vi "Scalar Field copy.vi"() -> ()   [LabVIEW 2017]
uses:
  <vilib>/Utility/sysdir.llb/System Directory Type.ctl
  <instrlib>/tio-labview/TIO Library/TIO Stream Open.vi
  <instrlib>/tio-labview/TIO Library/TIO RPC Send REQuest.vi
  <instrlib>/tio-labview/TIO Library/TIO RPC Blocking.vi
  <instrlib>/tio-labview/Labview Signal Processing/Log Binning.vi
  <instrlib>/tio-labview/TIO Library/TIO RPC Parse Reply.vi
  <instrlib>/tio-labview/TIO Library/TIO RPC Parse Reply Error.vi
  <instrlib>/tio-labview/TIO Library/TIO Data Stream Parse timebase Info.vi
  <instrlib>/tio-labview/TIO Library/TIO Data Stream Parse pstream Info.vi
  <instrlib>/tio-labview/TIO Library/TIO Data Stream Parse dstream Info.vi
  <instrlib>/tio-labview/TIO Library/TIO Serial Port Name Search.vi
  <instrlib>/tio-labview/TIO Library/TIO Stream Write.vi
  <instrlib>/tio-labview/TIO Library/TIO RPC Form Request.vi
  <instrlib>/tio-labview/TIO Library/TIO Stream Read.vi
  <instrlib>/tio-labview/Labview Signal Processing/Log Range.vi
  <instrlib>/tio-labview/TIO Library/TIO SLIP Serial Write.vi
  <instrlib>/tio-labview/TIO Library/TIO Form Packet.vi
  <instrlib>/tio-labview/TIO Library/TIO Parse Packet.vi
  <instrlib>/tio-labview/TIO Library/TIO SLIP Serial Read.vi
  <instrlib>/tio-labview/TIO Library/TIO SLIP Encode.vi
  <instrlib>/tio-labview/TIO Library/TIO Serial Checksum CRC32.vi
  <vilib>/Utility/tcp.llb/UDP Multicast Open.vi
  <vilib>/Utility/tcp.llb/UDP Multicast Read-Write Open.vi
  <instrlib>/tio-labview/TIO Library/TIO Serial Port Discovery.vi
  <vilib>/Instr/_visa.llb/VISA Configure Serial Port (Instr).vi
  <vilib>/Analysis/6fits.llb/General Polynomial Fit.vi
  <vilib>/measure/maspectr.llb/FFT Power Spectrum and PSD.vi
  <vilib>/measure/maspectr.llb/FFT Power Spectrum and PSD for 1 Chan.vi
  <instrlib>/tio-labview/TIO Library/TIO Stream Read Non-blocking.vi
panel:
  out "Signal":u8(slide) scale=0.0..256.0
  out "Status":T1(ring)
  in  "Reset":bool
  in  "URL":refnum<visa-resource-name>="tcp://localhost"
  in  "Quit":bool
  in  "Duration":dbl[unit]=1000.0
  out "A":T2(graph)
  in  "Log?":bool
  in  "Path":path
  in  "Clear C":bool
  in  "Save C":bool
  in  "Clear B":bool
  in  "Save B":bool
  in  "Clear A":bool
  in  "Save A":bool
  in  "Bin":bool=TRUE
  out "PSD":T3(graph)
  out "ID":string="Twinleaf VM4 R4"
  # "Field"
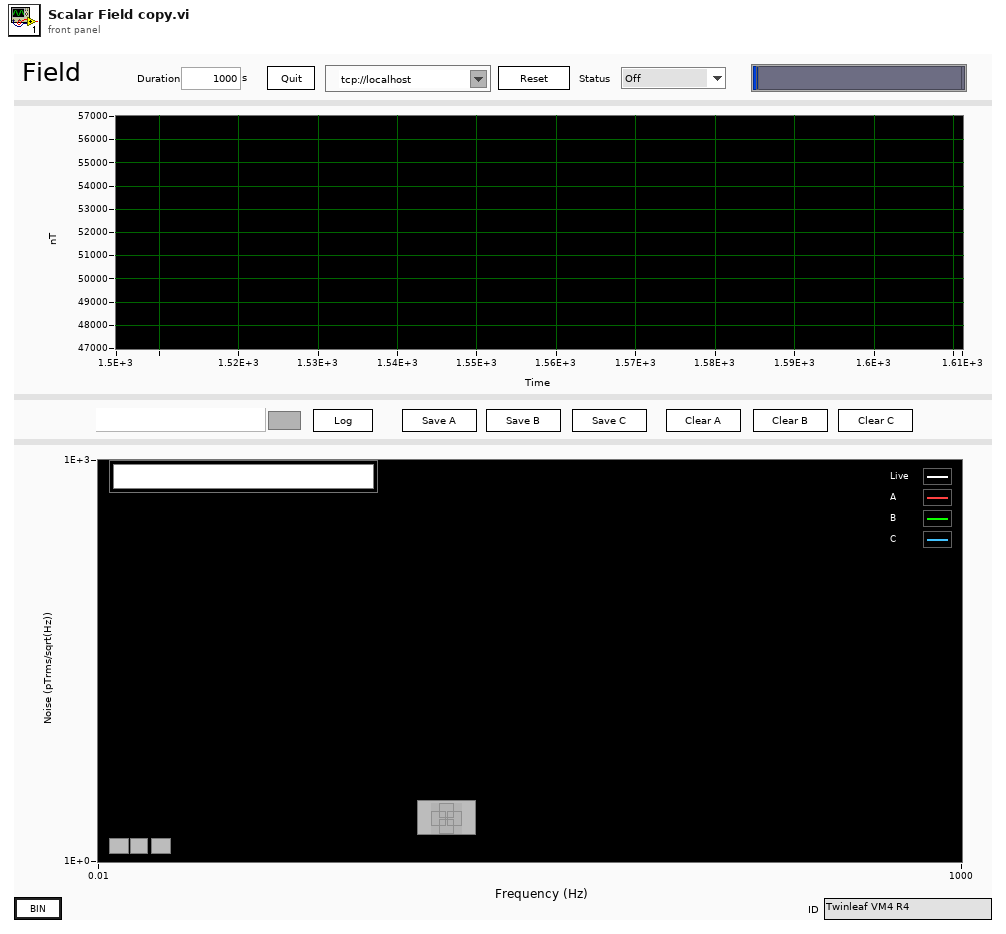
[diagram p1: front panel]
types:
  T1 = enum16{"Off", "Heating", "Laser", "Spin", "Locked"}
  T2 = cluster{"start":dbl, "dt":dbl, "Timeseries":dbl[]}
  T3 = cluster{"Frequencies Binned":dbl[], "Spectrum Binned":dbl[]}[]
  T4 = cluster{"Awaiting REP":bool, "REQ ID":u32, "dstreams in":cluster{"id":u16, "timebase id":u16, "period":u32, "offset":u32, "sample number":u64, "total components":u16, "flags":u16, "components":cluster{"pstream id":u16, "flags":u16, "period":u32, "offset":u32}[]}[], "pstreams":cluster{"id":u16, "timebase_id":u16, "period":u32, "offset":u32, "fmt":i32, "flags":u16, "channels":u16, "type":u8, "name":string, "column names":string[], "title":string, "units":string}[], "timebases":cluster{"id":u16, "source":u16, "epoch":u32, "start time":u32, "period numerator (µs)":i32, "period denominator (µs)":u16, "flags":u16, "stability":u8, "source id":string}[]}
  T5 = typedef "System Directory Type.ctl" = i32
  T6 = cluster{"TS Connection":cluster{"Type":enum16{"Serial", "TCP", "UDP", "mUDP"}, "URL":refnum<visa-resource-name>, "TO":u32, "Addr":u32, "Port":i32, "TCP":refnum<k5>, "UDP":refnum<k16>, "Route":string}, "REQ":refnum<queue>, "REP":refnum<queue>}
  T7 = cluster{"start":dbl, "dt":dbl, "Timeseries":sgl[][]}
  T8 = cluster{"dstream ID":u16, "Sample Number":u32, "Raw Data":string}
  T9 = cluster{"TC Connection":cluster{"Type":enum16{"Serial", "TCP", "UDP", "mUDP"}, "URL":refnum<visa-resource-name>, "TO":u32, "Addr":u32, "Port":i32, "TCP":refnum<k5>, "UDP":refnum<k16>, "Route":string}, "REQ":refnum<queue>, "REP":refnum<queue>}
  T10 = cluster{"start":dbl, "dt":dbl, "Timeseries":dbl[][]}
  T11 = cluster{"Name":string, "Waveform":cluster{"start":dbl, "dt":dbl, "Timeseries":dbl[][]}}[]
  T12 = cluster{"Frequencies Binned":dbl[], "Spectrum Binned":dbl[]}
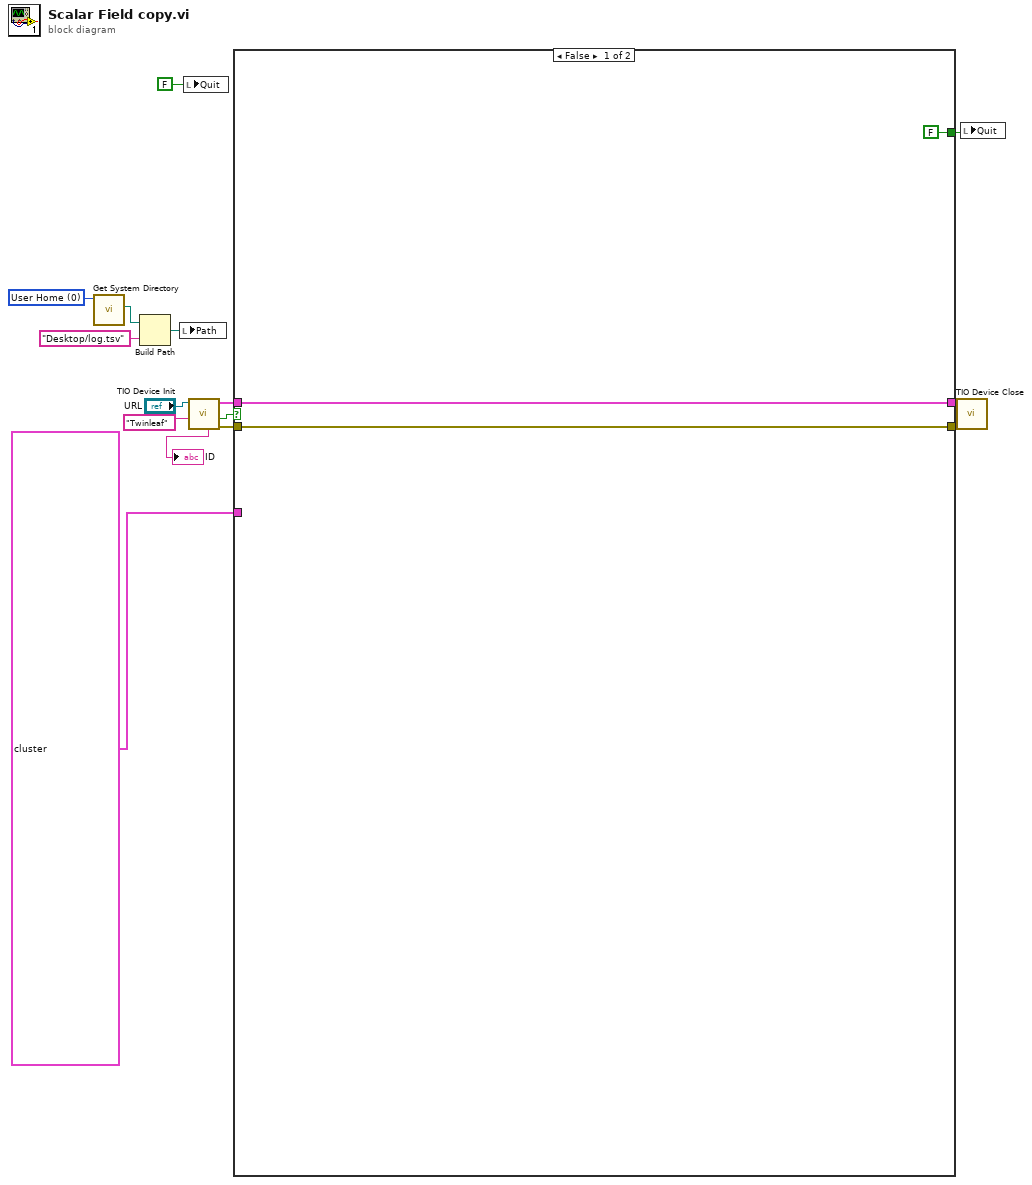
[diagram p0: block diagram]
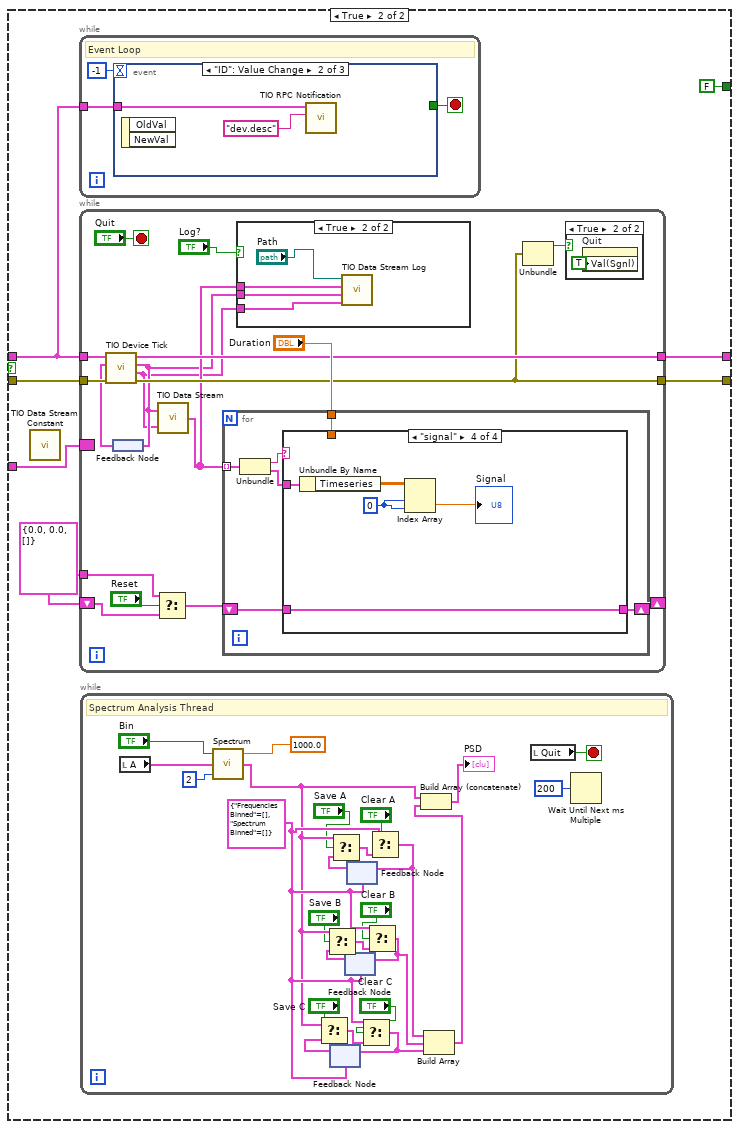
[diagram p2: hidden frame]
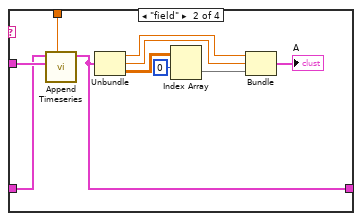
[diagram p6: hidden frame]
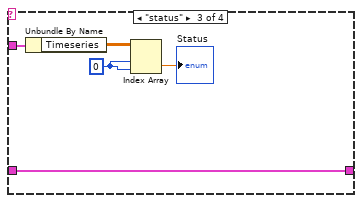
[diagram p7: hidden frame]
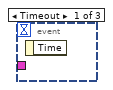
[diagram p8: hidden frame]
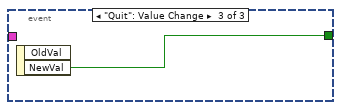
[diagram p9: hidden frame]
diagram:
  w8 = T5 0 items=["User Home"=0, "User Desktop"=1, "User Documents"=2, "User Application Data"=3, "User Preferences"=4, "User Temporary"=5, "Public Documents"=6, "Public Application Data"=7, "Public Preferences"=8, "Public Cache"=13, "System Core Libraries"=9, "System Installed Libraries"=10, "Application Files"=11, "Boot Volume Root"=12] ("system directory type")
  n1 = call <vilib>:"Get System Directory.vi"("system directory type"=w8) -> ("system directory"=w7:path)  [unwired: 10 in]
  n2 = Build Path(base path=w7, name or relative path="Desktop/log.tsv") -> (appended path=w5:path)
  n3 = local write "Path"(w5) -> ()
  n4 = local write "Quit"(FALSE ("Kill")) -> ()
  n5 = call <instrlib>:"TIO Device Init.vi"("ID"="Twinleaf" ("Prefix"), "URL"="URL") -> ("error out"=w14:errorcluster, "Connected"=w3:bool, "TIO"=w15:T6, "ID Verified"=→"ID":string)  [unwired: 5 in, 1 out]
  n6 = case shown="False" w3 {
    tunnel: w15 -> [w18 w24]
    tunnel: w14 -> [w17 w25]
    tunnel: [w17 w22] -> w10
    tunnel: [w18 w21] -> w9
    tunnel: T4 {"Awaiting REP"=FALSE, "REQ ID"=500, "dstreams in"=[{"id"=0, "timebase id"=1, "period"=16, "offset"=0, "sample number"=10656, "total components"=6, "flags"=1, "components"=[{"pstream id"=0, "flags"=0, "period"=1, "offset"=0}, {"pstream id"=1, "flags"=1, "period"=1, "offset"=0}, {"pstream id"=32770, "flags"=0, "period"=8, "offset"=0}, {"pstream id"=32772, "flags"=0, "period"=8, "offset"=0}, {"pstream id"=32774, "flags"=1, "period"=64, "offset"=0}, {"pstream id"=2, "flags"=1, "period"=64, "offset"=0}]}, {"id"=0, "timebase id"=0, "period"=0, "offset"=0, "sample number"=0, "total components"=0, "flags"=0, "components"=[]}, {"id"=0, "timebase id"=0, "period"=0, "offset"=0, "sample number"=0, "total components"=0, "flags"=0, "components"=[]}, {"id"=0, "timebase id"=0, "period"=0, "offset"=0, "sample number"=0, "total components"=0, "flags"=0, "components"=[]}, {"id"=0, "timebase id"=0, "period"=0, "offset"=0, "sample number"=0, "total components"=0, "flags"=0, "components"=[]}, {"id"=0, "timebase id"=0, "period"=0, "offset"=0, "sample number"=0, "total components"=0, "flags"=0, "components"=[]}, {"id"=0, "timebase id"=0, "period"=0, "offset"=0, "sample number"=0, "total components"=0, "flags"=0, "components"=[]}, {"id"=0, "timebase id"=0, "period"=0, "offset"=0, "sample number"=0, "total components"=0, "flags"=0, "components"=[]}, {"id"=0, "timebase id"=0, "period"=0, "offset"=0, "sample number"=0, "total components"=0, "flags"=0, "components"=[]}, {"id"=0, "timebase id"=0, "period"=0, "offset"=0, "sample number"=0, "total components"=0, "flags"=0, "components"=[]}, {"id"=0, "timebase id"=0, "period"=0, "offset"=0, "sample number"=0, "total components"=0, "flags"=0, "components"=[]}, {"id"=0, "timebase id"=0, "period"=0, "offset"=0, "sample number"=0, "total components"=0, "flags"=0, "components"=[]}, {"id"=0, "timebase id"=0, "period"=0, "offset"=0, "sample number"=0, "total components"=0, "flags"=0, "components"=[]}, {"id"=0, "timebase id"=0, "period"=0, "offset"=0, "sample number"=0, "total components"=0, "flags"=0, "components"=[]}, {"id"=0, "timebase id"=0, "period"=0, "offset"=0, "sample number"=0, "total components"=0, "flags"=0, "components"=[]}, {"id"=0, "timebase id"=0, "period"=0, "offset"=0, "sample number"=0, "total components"=0, "flags"=0, "components"=[]}, {"id"=0, "timebase id"=0, "period"=0, "offset"=0, "sample number"=0, "total components"=0, "flags"=0, "components"=[]}, {"id"=0, "timebase id"=0, "period"=0, "offset"=0, "sample number"=0, "total components"=0, "flags"=0, "components"=[]}, {"id"=0, "timebase id"=0, "period"=0, "offset"=0, "sample number"=0, "total components"=0, "flags"=0, "components"=[]}, {"id"=0, "timebase id"=0, "period"=0, "offset"=0, "sample number"=0, "total components"=0, "flags"=0, "components"=[]}, {"id"=0, "timebase id"=0, "period"=0, "offset"=0, "sample number"=0, "total components"=0, "flags"=0, "components"=[]}, {"id"=0, "timebase id"=0, "period"=0, "offset"=0, "sample number"=0, "total components"=0, "flags"=0, "components"=[]}, {"id"=0, "timebase id"=0, "period"=0, "offset"=0, "sample number"=0, "total components"=0, "flags"=0, "components"=[]}, {"id"=0, "timebase id"=0, "period"=0, "offset"=0, "sample number"=0, "total components"=0, "flags"=0, "components"=[]}, {"id"=0, "timebase id"=0, "period"=0, "offset"=0, "sample number"=0, "total components"=0, "flags"=0, "components"=[]}, {"id"=0, "timebase id"=0, "period"=0, "offset"=0, "sample number"=0, "total components"=0, "flags"=0, "components"=[]}, {"id"=0, "timebase id"=0, "period"=0, "offset"=0, "sample number"=0, "total components"=0, "flags"=0, "components"=[]}, {"id"=0, "timebase id"=0, "period"=0, "offset"=0, "sample number"=0, "total components"=0, "flags"=0, "components"=[]}, {"id"=0, "timebase id"=0, "period"=0, "offset"=0, "sample number"=0, "total components"=0, "flags"=0, "components"=[]}, {"id"=0, "timebase id"=0, "period"=0, "offset"=0, "sample number"=0, "total components"=0, "flags"=0, "components"=[]}, {"id"=0, "timebase id"=0, "period"=0, "offset"=0, "sample number"=0, "total components"=0, "flags"=0, "components"=[]}, {"id"=0, "timebase id"=0, "period"=0, "offset"=0, "sample number"=0, "total components"=0, "flags"=0, "components"=[]}], "pstreams"=[{"id"=0, "timebase_id"=1, "period"=8, "offset"=0, "fmt"=-1, "flags"=0, "channels"=1, "type"=66, "name"="field", "column names"=["B"], "title"="Magnetic field", "units"="nT"}, {"id"=1, "timebase_id"=0, "period"=1, "offset"=0, "fmt"=-1, "flags"=0, "channels"=1, "type"=16, "name"="signal", "column names"=[""], "title"="Signal", "units"=""}, {"id"=2, "timebase_id"=0, "period"=1, "offset"=0, "fmt"=-1, "flags"=0, "channels"=1, "type"=16, "name"="status", "column names"=[""], "title"="Status", "units"=""}, {"id"=0, "timebase_id"=0, "period"=0, "offset"=0, "fmt"=0, "flags"=0, "channels"=0, "type"=0, "name"="", "column names"=[], "title"="", "units"=""}, {"id"=0, "timebase_id"=0, "period"=0, "offset"=0, "fmt"=0, "flags"=0, "channels"=0, "type"=0, "name"="", "column names"=[], "title"="", "units"=""}, {"id"=0, "timebase_id"=0, "period"=0, "offset"=0, "fmt"=0, "flags"=0, "channels"=0, "type"=0, "name"="", "column names"=[], "title"="", "units"=""}, {"id"=0, "timebase_id"=0, "period"=0, "offset"=0, "fmt"=0, "flags"=0, "channels"=0, "type"=0, "name"="", "column names"=[], "title"="", "units"=""}, {"id"=0, "timebase_id"=0, "period"=0, "offset"=0, "fmt"=0, "flags"=0, "channels"=0, "type"=0, "name"="", "column names"=[], "title"="", "units"=""}, {"id"=0, "timebase_id"=0, "period"=0, "offset"=0, "fmt"=0, "flags"=0, "channels"=0, "type"=0, "name"="", "column names"=[], "title"="", "units"=""}, {"id"=0, "timebase_id"=0, "period"=0, "offset"=0, "fmt"=0, "flags"=0, "channels"=0, "type"=0, "name"="", "column names"=[], "title"="", "units"=""}, {"id"=0, "timebase_id"=0, "period"=0, "offset"=0, "fmt"=0, "flags"=0, "channels"=0, "type"=0, "name"="", "column names"=[], "title"="", "units"=""}, {"id"=0, "timebase_id"=0, "period"=0, "offset"=0, "fmt"=0, "flags"=0, "channels"=0, "type"=0, "name"="", "column names"=[], "title"="", "units"=""}, {"id"=0, "timebase_id"=0, "period"=0, "offset"=0, "fmt"=0, "flags"=0, "channels"=0, "type"=0, "name"="", "column names"=[], "title"="", "units"=""}, {"id"=0, "timebase_id"=0, "period"=0, "offset"=0, "fmt"=0, "flags"=0, "channels"=0, "type"=0, "name"="", "column names"=[], "title"="", "units"=""}, {"id"=0, "timebase_id"=0, "period"=0, "offset"=0, "fmt"=0, "flags"=0, "channels"=0, "type"=0, "name"="", "column names"=[], "title"="", "units"=""}, {"id"=0, "timebase_id"=0, "period"=0, "offset"=0, "fmt"=0, "flags"=0, "channels"=0, "type"=0, "name"="", "column names"=[], "title"="", "units"=""}, {"id"=32768, "timebase_id"=1, "period"=8, "offset"=0, "fmt"=-1, "flags"=0, "channels"=1, "type"=66, "name"="_field.raw", "column names"=["B"], "title"="Magnetic field", "units"="nT"}, {"id"=32769, "timebase_id"=1, "period"=8, "offset"=0, "fmt"=-1, "flags"=0, "channels"=3, "type"=66, "name"="_spin.raw", "column names"=["measure", "reference", "output"], "title"="Spin lock", "units"=""}, {"id"=32770, "timebase_id"=1, "period"=8, "offset"=0, "fmt"=-1, "flags"=0, "channels"=3, "type"=66, "name"="spin", "column names"=["measure", "reference", "output"], "title"="Spin lock", "units"=""}, {"id"=32771, "timebase_id"=1, "period"=2, "offset"=0, "fmt"=-1, "flags"=0, "channels"=3, "type"=66, "name"="_laser.raw", "column names"=["measure", "reference", "output"], "title"="Laser lock", "units"=""}, {"id"=32772, "timebase_id"=1, "period"=2, "offset"=0, "fmt"=-1, "flags"=0, "channels"=3, "type"=66, "name"="laser", "column names"=["measure", "reference", "output"], "title"="Laser lock", "units"=""}, {"id"=32773, "timebase_id"=2, "period"=1, "offset"=0, "fmt"=-1, "flags"=0, "channels"=3, "type"=66, "name"="_therm.raw", "column names"=["measure", "reference", "output"], "title"="Cell temperature", "units"="°C"}, {"id"=32774, "timebase_id"=2, "period"=1, "offset"=0, "fmt"=-1, "flags"=0, "channels"=3, "type"=66, "name"="therm", "column names"=["measure", "reference", "output"], "title"="Cell temperature", "units"="°C"}, {"id"=32775, "timebase_id"=0, "period"=1, "offset"=0, "fmt"=-1, "flags"=0, "channels"=1, "type"=66, "name"="_cpu.raw", "column names"=[""], "title"="CPU load", "units"="%"}, {"id"=32776, "timebase_id"=0, "period"=1, "offset"=0, "fmt"=-1, "flags"=0, "channels"=1, "type"=66, "name"="cpu", "column names"=[""], "title"="CPU load", "units"="%"}, {"id"=0, "timebase_id"=0, "period"=0, "offset"=0, "fmt"=0, "flags"=0, "channels"=0, "type"=0, "name"="", "column names"=[], "title"="", "units"=""}, {"id"=0, "timebase_id"=0, "period"=0, "offset"=0, "fmt"=0, "flags"=0, "channels"=0, "type"=0, "name"="", "column names"=[], "title"="", "units"=""}, {"id"=0, "timebase_id"=0, "period"=0, "offset"=0, "fmt"=0, "flags"=0, "channels"=0, "type"=0, "name"="", "column names"=[], "title"="", "units"=""}, {"id"=0, "timebase_id"=0, "period"=0, "offset"=0, "fmt"=0, "flags"=0, "channels"=0, "type"=0, "name"="", "column names"=[], "title"="", "units"=""}, {"id"=0, "timebase_id"=0, "period"=0, "offset"=0, "fmt"=0, "flags"=0, "channels"=0, "type"=0, "name"="", "column names"=[], "title"="", "units"=""}, {"id"=0, "timebase_id"=0, "period"=0, "offset"=0, "fmt"=0, "flags"=0, "channels"=0, "type"=0, "name"="", "column names"=[], "title"="", "units"=""}, {"id"=0, "timebase_id"=0, "period"=0, "offset"=0, "fmt"=0, "flags"=0, "channels"=0, "type"=0, "name"="", "column names"=[], "title"="", "units"=""}], "timebases"=[{"id"=0, "source"=513, "epoch"=0, "start time"=0, "period numerator (µs)"=100000000, "period denominator (µs)"=1000, "flags"=0, "stability"=1, "source id"="\u0000\u0000\u0000\u0000\u0000À\u0001\u0000\u0000\u0000@\u0000\u001f\u0000\u0011P6W462 "}, {"id"=1, "source"=513, "epoch"=187833658, "start time"=0, "period numerator (µs)"=312500, "period denominator (µs)"=1000, "flags"=0, "stability"=1, "source id"="\u0000\u0000\u0000¬Å'7\u0001\u0000\u0000\u0000@\u0000\u001f\u0000\u0011P6W462 "}, {"id"=2, "source"=513, "epoch"=62622070, "start time"=0, "period numerator (µs)"=125000000, "period denominator (µs)"=1000, "flags"=0, "stability"=1, "source id"="\u0000\u0000\u0000\nף;\u0001\u0000\u0000\u0000@\u0000\u001f\u0000\u0011P6W462 "}, {"id"=0, "source"=0, "epoch"=0, "start time"=0, "period numerator (µs)"=0, "period denominator (µs)"=0, "flags"=0, "stability"=0, "source id"=""}, {"id"=0, "source"=0, "epoch"=0, "start time"=0, "period numerator (µs)"=0, "period denominator (µs)"=0, "flags"=0, "stability"=0, "source id"=""}, {"id"=0, "source"=0, "epoch"=0, "start time"=0, "period numerator (µs)"=0, "period denominator (µs)"=0, "flags"=0, "stability"=0, "source id"=""}, {"id"=0, "source"=0, "epoch"=0, "start time"=0, "period numerator (µs)"=0, "period denominator (µs)"=0, "flags"=0, "stability"=0, "source id"=""}, {"id"=0, "source"=0, "epoch"=0, "start time"=0, "period numerator (µs)"=0, "period denominator (µs)"=0, "flags"=0, "stability"=0, "source id"=""}, {"id"=0, "source"=0, "epoch"=0, "start time"=0, "period numerator (µs)"=0, "period denominator (µs)"=0, "flags"=0, "stability"=0, "source id"=""}, {"id"=0, "source"=0, "epoch"=0, "start time"=0, "period numerator (µs)"=0, "period denominator (µs)"=0, "flags"=0, "stability"=0, "source id"=""}, {"id"=0, "source"=0, "epoch"=0, "start time"=0, "period numerator (µs)"=0, "period denominator (µs)"=0, "flags"=0, "stability"=0, "source id"=""}, {"id"=0, "source"=0, "epoch"=0, "start time"=0, "period numerator (µs)"=0, "period denominator (µs)"=0, "flags"=0, "stability"=0, "source id"=""}, {"id"=0, "source"=0, "epoch"=0, "start time"=0, "period numerator (µs)"=0, "period denominator (µs)"=0, "flags"=0, "stability"=0, "source id"=""}, {"id"=0, "source"=0, "epoch"=0, "start time"=0, "period numerator (µs)"=0, "period denominator (µs)"=0, "flags"=0, "stability"=0, "source id"=""}, {"id"=0, "source"=0, "epoch"=0, "start time"=0, "period numerator (µs)"=0, "period denominator (µs)"=0, "flags"=0, "stability"=0, "source id"=""}, {"id"=0, "source"=0, "epoch"=0, "start time"=0, "period numerator (µs)"=0, "period denominator (µs)"=0, "flags"=0, "stability"=0, "source id"=""}, {"id"=0, "source"=0, "epoch"=0, "start time"=0, "period numerator (µs)"=0, "period denominator (µs)"=0, "flags"=0, "stability"=0, "source id"=""}, {"id"=0, "source"=0, "epoch"=0, "start time"=0, "period numerator (µs)"=0, "period denominator (µs)"=0, "flags"=0, "stability"=0, "source id"=""}, {"id"=0, "source"=0, "epoch"=0, "start time"=0, "period numerator (µs)"=0, "period denominator (µs)"=0, "flags"=0, "stability"=0, "source id"=""}, {"id"=0, "source"=0, "epoch"=0, "start time"=0, "period numerator (µs)"=0, "period denominator (µs)"=0, "flags"=0, "stability"=0, "source id"=""}, {"id"=0, "source"=0, "epoch"=0, "start time"=0, "period numerator (µs)"=0, "period denominator (µs)"=0, "flags"=0, "stability"=0, "source id"=""}, {"id"=0, "source"=0, "epoch"=0, "start time"=0, "period numerator (µs)"=0, "period denominator (µs)"=0, "flags"=0, "stability"=0, "source id"=""}, {"id"=0, "source"=0, "epoch"=0, "start time"=0, "period numerator (µs)"=0, "period denominator (µs)"=0, "flags"=0, "stability"=0, "source id"=""}, {"id"=0, "source"=0, "epoch"=0, "start time"=0, "period numerator (µs)"=0, "period denominator (µs)"=0, "flags"=0, "stability"=0, "source id"=""}, {"id"=0, "source"=0, "epoch"=0, "start time"=0, "period numerator (µs)"=0, "period denominator (µs)"=0, "flags"=0, "stability"=0, "source id"=""}, {"id"=0, "source"=0, "epoch"=0, "start time"=0, "period numerator (µs)"=0, "period denominator (µs)"=0, "flags"=0, "stability"=0, "source id"=""}, {"id"=0, "source"=0, "epoch"=0, "start time"=0, "period numerator (µs)"=0, "period denominator (µs)"=0, "flags"=0, "stability"=0, "source id"=""}, {"id"=0, "source"=0, "epoch"=0, "start time"=0, "period numerator (µs)"=0, "period denominator (µs)"=0, "flags"=0, "stability"=0, "source id"=""}, {"id"=0, "source"=0, "epoch"=0, "start time"=0, "period numerator (µs)"=0, "period denominator (µs)"=0, "flags"=0, "stability"=0, "source id"=""}, {"id"=0, "source"=0, "epoch"=0, "start time"=0, "period numerator (µs)"=0, "period denominator (µs)"=0, "flags"=0, "stability"=0, "source id"=""}, {"id"=0, "source"=0, "epoch"=0, "start time"=0, "period numerator (µs)"=0, "period denominator (µs)"=0, "flags"=0, "stability"=0, "source id"=""}, {"id"=0, "source"=0, "epoch"=0, "start time"=0, "period numerator (µs)"=0, "period denominator (µs)"=0, "flags"=0, "stability"=0, "source id"=""}]} ("TIO State") -> [_ w20]
    tunnel: [FALSE ("Kill") FALSE ("Kill")] -> w1
    frame False {
    }
    frame True {
      w23 = T7 {"start"=0.0, "dt"=0.0, "Timeseries"=[]}
      n7 = call <instrlib>:"TIO Data Stream Constant.vi"() -> ()  [unwired: 1 out]
      n8 = while {
        tunnel: w24 -> [w76]
        stop <- w75 stop-if-true
        # "Event Loop"
        n9 = event shown="[1] \"ID\": Value Change" {
          selector: _ -> [_ _ _]
          dyn-events: _ -> [_ _ _]
          timeout: -1 -> [_ _ _]
          tunnel: w76 -> [_ w79 _]
          tunnel: [_ _ w80] -> w75
          event Timeout {
            n10 = event-data() -> ()  [unwired: 1 in, 1 out]
          }
          event "ID": Value Change {
            n11 = event-data() -> ()  [unwired: 1 in, 2 out]
            n12 = call <instrlib>:"TIO RPC Notification.vi"("Topic"="dev.desc", "TIO"=w79) -> ()  [unwired: 6 in, 3 out]
          }
          event "Quit": Value Change {
            n13 = event-data() -> ("NewVal"=w80:bool)  [unwired: 1 in, 1 out]
          }
        }
      }
      n14 = while {
        tunnel: w24 -> [w42]
        tunnel: w25 -> [w41]
        shift-right: [w38] -> _
        shift-left: w23 -> [w36]
        tunnel: [w31] -> w22
        border: w20 -> [_]
        tunnel: w23 -> [w34]
        tunnel: [w32] -> w21
        stop <- "Quit" stop-if-true
        n15 = feedback #1() -> (w37:T4)
        n16 = call <instrlib>:"TIO Device Tick.vi"("Error in"=w41, "TIO State"=w37, "TIO"=w42) -> ("Error out"=w31:errorcluster, "Data Out"=w27:T8, "TIO State"=w28:T4, "TIO"=w32:T9)  [unwired: 5 in]
        n17 = feedback-in #1(w28) -> ()
        n18 = Select(t=w34, s="Reset", f=w36) -> (s? t:f=w35:T10)
        n19 = call <instrlib>:"TIO Data Stream.vi"("Raw Data"=w27, "TIO State"=w28) -> ("Data Out"=w29:T11)
        n20 = for {
          tunnel: "Duration" -> [w53]
          tunnel: w29 -> [w50] mode=indexing
          shift-right: [w52] -> w38
          shift-left: w35 -> [w51]
          n21 = Unbundle(w50) -> ("Name"=w49:string, "Waveform"=w48:T10)
          n22 = case shown="\"signal\"" w49 {
            tunnel: w53 -> [_ w64 _ _]
            tunnel: w48 -> [_ w58 w69 w74]
            tunnel: [w54 w57 w65 w71] -> w52
            tunnel: w51 -> [w54 w56 w65 w71]
            frame Default {
            }
            frame "field" {
              n23 = call <instrlib>:"Append Timeseries.vi"("Duration"=w64, "In New"=w58, "In Old"=w56) -> ("Appended"=w57:T10)  [unwired: 8 in]
              n24 = Unbundle(w57) -> ("start"=w63:dbl, "dt"=w61:dbl, "Timeseries"=w59:dbl[][])
              n25 = Index Array(array=w59, index (row)=0 ("disabled index (col)")) -> (element=w55:dbl[])  [unwired: 1 in]
              n26 = Bundle("start"=w63, "dt"=w61, "Timeseries"=w55) -> (→"A":T2)  [unwired: 1 in]
            }
            frame "status" {
              w67 = 0 ("disabled index (col)")
              n27 = Unbundle By Name(w69) -> ("Timeseries"=w68:dbl[][])
              n28 = Index Array(array=w68, index (row)=w67, index (col)=w67) -> (element=→"Status":dbl)
            }
            frame "signal" {
              w72 = 0 ("disabled index (col)")
              n29 = Unbundle By Name(w74) -> ("Timeseries"=w73:dbl[][])
              n30 = Index Array(array=w73, index (row)=w72, index (col)=w72) -> (element=→"Signal":dbl)
            }
          }
        }
        n31 = case shown="True" "Log?" {
          tunnel: w29 -> [_ w46]
          tunnel: w28 -> [_ w45]
          tunnel: w27 -> [_ w44]
          frame False {
          }
          frame True {
            n32 = call <instrlib>:"TIO Data Stream Log.vi"(8:"Data Out"=w44, "TIO State"=w45, 10:"Data Out"=w46, "Log to file"="Path") -> ()  [unwired: 8 in]
          }
        }
        n33 = Unbundle(w31) -> ("status"=w30:bool)  [unwired: 2 out]
        n34 = case shown="True" w30 {
          frame False {
          }
          frame True {
            n35 = property on="Quit" class="Bool (strict)"("Val(Sgnl)"=TRUE ("Value (Signaling)")) -> ()  [unwired: 2 in, 2 out]
          }
        }
      }
      n36 = while {
        stop <- w103 stop-if-true
        w90 = T12 {"Frequencies Binned"=[], "Spectrum Binned"=[]} ("Cluster")
        # "Spectrum Analysis Thread"
        n37 = local read "A"() -> (w102:T2)
        n38 = call <instrlib>:"Spectrum.vi"("Gain"=1000.0, "Remove Polynomial Order"=2, "Waveform 1"=w102, "Binning"="Bin") -> ("Cluster"=w87:T12)  [unwired: 1 in]
        n39 = feedback #2(w90) -> (w96:T12)
        n40 = Select(t=w87, s="Save C", f=w96) -> (s? t:f=w97:T12)
        n41 = feedback #3(w90) -> (w95:T12)
        n42 = Select(t=w87, s="Save B", f=w95) -> (s? t:f=w94:T12)
        n43 = feedback #4(w90) -> (w92:T12)
        n44 = Select(t=w87, s="Save A", f=w92) -> (s? t:f=w93:T12)
        n45 = Select(t=w90, s="Clear C", f=w97) -> (s? t:f=w89:T12)
        n46 = feedback-in #2(w89) -> ()
        n47 = Select(t=w90, s="Clear B", f=w94) -> (s? t:f=w98:T12)
        n48 = feedback-in #3(w98) -> ()
        n49 = Select(t=w90, s="Clear A", f=w93) -> (s? t:f=w99:T12)
        n50 = feedback-in #4(w99) -> ()
        n51 = Build Array(w99, w98, w89) -> (w91:T3)
        n52 = Build Array (concatenate)(w87, w91) -> (→"PSD":T3)
        n53 = local read "Quit"() -> (w103:bool)
        n54 = Wait Until Next ms Multiple(millisecond multiple=u32 200) -> ()  [unwired: 1 out]
      }
    }
  }
  n55 = call <instrlib>:"TIO Device Close.vi"("Error in"=w10, "TIO"=w9) -> ()  [unwired: 10 in]
  n56 = local write "Quit"(w1) -> ()
